vi "Set Node State.vi"(8 "Error In":errorcluster, 10 "CANopen Message":refnum<class "CANopen Response Message.lvclass">, 11 "reference in":refnum<class "Network Mangement.lvclass">) -> (0 "Error Out":errorcluster, 2 "New Node/State?":bool, 3 "reference out":refnum<class "Network Mangement.lvclass">)   [LabVIEW 2024, in "Network Mangement.lvclass"]
uses:
  Network Mangement.lvclass
  CANopen Response/CANopen Response Message.lvclass
  source/CANopen Message/CANopen Message.lvclass
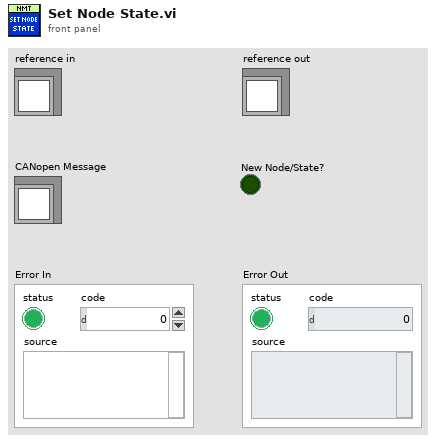
[diagram p1: front panel]
types:
  T1 = typedef "CANopen Response Message.lvclass/Server Command Specifier.ctl" = enum8{"Upload Segment Response", "Download Segment Response", "Initiate Upload Response", "Initiate Download Response", "Heartbeat", "Block Download"}
  T2 = typedef "Network Mangement.lvclass/ObjectAttributes.ctl" = cluster{"Nodes":map{u8, u8}, "Heartbeats":map{u8, cluster{"Period":u16, "Timeout":u16, "Last Beat":timestamp}}, "Events":cluster{"Stop Heartbeat Checker":refnum<user-event>, "Heartbeat Timeout":refnum<user-event>, "Heartbeat Checker Error":refnum<user-event>}, "Heartbeat Checker":refnum<vi>}
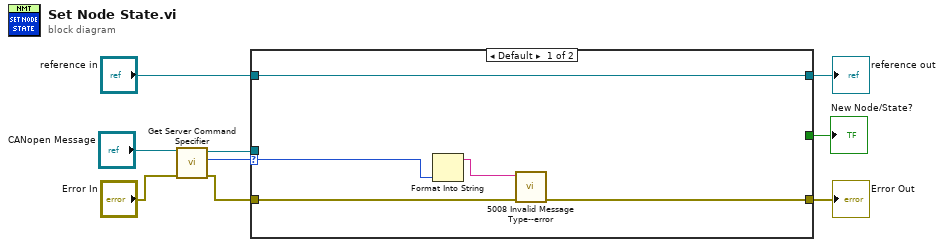
[diagram p0: block diagram]
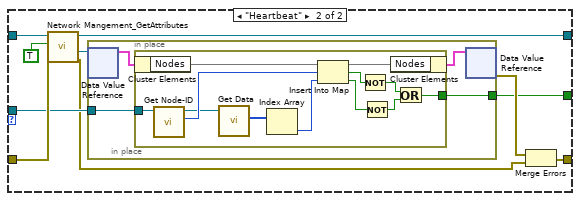
[diagram p2: hidden frame]
diagram:
  n1 = call-dynamic "Get Server Command Specifier.vi"("error in"="Error In", "CANopen Response in"="CANopen Message") -> ("error out"=w3:errorcluster, "Server Command Specifier"=w2:T1, "CANopen Response out"=w5:refnum<class "CANopen Response Message.lvclass">)  [unwired: 7 in]
  n2 = case shown="Default" w2 {
    selector: w2 -> [w10 _]
    tunnel: w3 -> [w13 w24]
    tunnel: [w12 w23] -> w9
    tunnel: "reference in" -> [w14 w22]
    tunnel: [w14 w21] -> w7
    tunnel: w5 -> [_ w17]
    tunnel: [_ w16] -> w1
    frame Default {
      n3 = Format Into String(w10) -> (resulting string=w11:string)  [unwired: 3 in, 1 out]
      n4 = call "5008 Invalid Message Type--error.vi"("error in"=w13, "Argument"=w11) -> ("error out"=w12:errorcluster)  [unwired: 9 in]
    }
    frame "Heartbeat" {
      n5 = call "Network Mangement_GetAttributes.vi"("Error In"=w24, "OnlyGetDvrReference(False)"=TRUE, "reference in"=w22) -> ("Error Out"=w15:errorcluster, "DataRef"=w19:refnum<data-value>, "reference out"=w21:refnum<class "Network Mangement.lvclass">)  [unwired: 5 in, 1 out]
      n6 = in-place {
        in-place-border: w17 -> [w27]
        in-place-border: [w25] -> w16
        n7 = in-place-dvr #1(w19) -> (w28:T2)  [unwired: 1 out]
        n8 = in-place {
          in-place-border: w27 -> [w38]
          in-place-border: [w31] -> w25
          n9 = in-place-cluster #2(w28) -> ("Nodes"=w40:map{u8, u8})
          n10 = call "Get Node-ID.vi"("CANopen Message in"=w38) -> ("Node-ID"=w37:u8, "CANopen Message out"=w36:refnum<class "CANopen Response Message.lvclass">)  [unwired: 8 in, 1 out]
          n11 = call "Get Data.vi"("CANopen Message in"=w36) -> ("Data"=w35:u8[])  [unwired: 8 in, 2 out]
          n12 = Index Array(array=w35) -> (element=w33:u8)  [unwired: 1 in]
          n13 = Insert Into Map(map in=w40, key=w37, value=w33) -> (map out=w39:map{u8, u8}, key already included?=w34:bool, value unchanged?=w29:bool)
          n14 = Not(x=w34) -> (.not. x?=w32:bool)
          n15 = Not(x=w29) -> (.not. x?=w30:bool)
          n16 = in-place-cluster #2("Nodes"=w39) -> (w26:T2)
          n17 = Or(x=w32, y=w30) -> (x .or. y?=w31:bool)
        }
        n18 = in-place-dvr #1(w26) -> (w18:errorcluster)  [unwired: 1 out]
      }
      n19 = Merge Errors(w18, w15) -> (w23:errorcluster)
    }
  }
  "Error Out" <- w9
  "reference out" <- w7
  "New Node/State?" <- w1
